vi "solar_misc Create Project Tree.vi"(8 "error in (no error)":errorcluster, 10 "Project Tree":refnum<vi>, 11 "Project (*.lvproj)":path) -> (0 "error out":errorcluster, 2 "My Computer":refnum<vi>, 3 "Project":refnum<vi>, 5 "App Ref":refnum<vi>)   [LabVIEW 2018]
doc: "This utility displays a project's items view in a tree control. Useful for scripting."
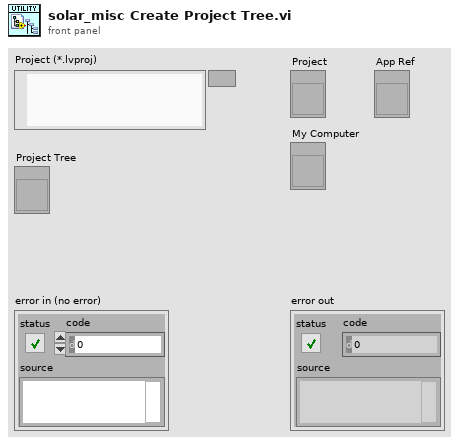
[diagram p1: front panel]
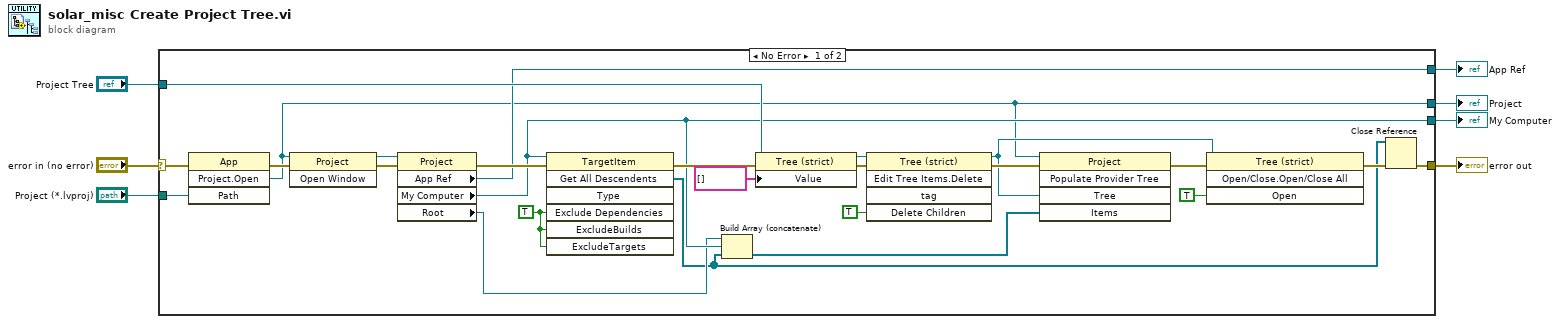
[diagram p0: block diagram]
diagram:
  n1 = case shown="No Error" "error in (no error)" {
    selector: "error in (no error)" -> [w25 w33]
    tunnel: "Project (*.lvproj)" -> [w32 _]
    tunnel: [w12 _] -> w6
    tunnel: [w16 _] -> w5
    tunnel: "Project Tree" -> [w22 _]
    tunnel: [w24 w33] -> w2
    tunnel: [w19 _] -> w1
    frame No Error {
      w8 = TRUE ("ExcludeDependencies")
      n2 = invoke class="App" method="Project.Open"(error in=w25, "Path"=w32) -> (error out=w30:errorcluster, "Project:Open"=w12:refnum<vi>)  [unwired: 2 in, 2 out]
      n3 = invoke class="Project" method="Open Window"(reference=w12, error in=w30) -> (reference out=w11:refnum<vi>, error out=w13:errorcluster)  [unwired: 1 in, 1 out]
      n4 = property class="Project"(reference=w11, error in=w13) -> (error out=w29:errorcluster, "App Ref"=w19:refnum<vi>, "My Computer"=w16:refnum<vi>, "Root"=w10:refnum<vi>)  [unwired: 1 out]
      n5 = invoke class="TargetItem" method="Get All Descendents"(reference=w16, error in=w29, "Exclude Dependencies"=w8, "ExcludeBuilds"=w8, "ExcludeTargets"=w8) -> (error out=w18:errorcluster, "All Descendents"=w9:refnum<vi>[])  [unwired: 2 in, 5 out]
      n6 = Build Array (concatenate)(w10, w16, w9) -> (w15:refnum<vi>[])
      n7 = property class="Tree (strict)"(reference=w22, error in=w18, "Value"=string[] []) -> (reference out=w21:refnum<vi>, error out=w23:errorcluster)
      n8 = invoke class="Tree (strict)" method="Edit Tree Items.Delete"(reference=w21, error in=w23, "Delete Children"=TRUE ("Delete Children?")) -> (reference out=w17:refnum<vi>, error out=w27:errorcluster)  [unwired: 2 in, 3 out]
      n9 = invoke class="Project" method="Populate Provider Tree"(reference=w12, error in=w27, "Tree"=w17, "Items"=w15) -> (error out=w31:errorcluster)  [unwired: 1 in, 4 out]
      n10 = invoke class="Tree (strict)" method="Open/Close.Open/Close All"(reference=w17, error in=w31, "Open"=TRUE ("Open?")) -> (error out=w14:errorcluster)  [unwired: 1 in, 3 out]
      n11 = Close Reference(reference=w9, error in (no error)=w14) -> (error out=w24:errorcluster)
    }
    frame Error {
    }
  }
  "error out" <- w2
  "Project" <- w6
  "My Computer" <- w5
  "App Ref" <- w1
